vi "Find #SameModeChild.vi"(6 "Stop Traverse Child":bool, 8 "error in":errorcluster caption="错误输入（无错误）", 9 "Data in":cluster{"Split Mode":i32, "#sameMode":i32}={"Split Mode"=-1, "#sameMode"=0}, 11 "PanelRootNode.lvclass":refnum<class "PanelRootNode.lvclass">) -> (0 "error out":errorcluster caption="错误输出", 1 "Data out":cluster{"Split Mode":i32, "#sameMode":i32}, 3 "PanelRootNode.lvclass 2":refnum<class "PanelRootNode.lvclass">)   [LabVIEW 2013, in "PanelRootNode.lvclass"]
uses:
  PanelRootNode.lvclass
  PanelLinkNode/PanelLinkNode.lvclass/PanelLinkNode.ctl
  PanelLinkNode/PanelLinkNode.lvclass
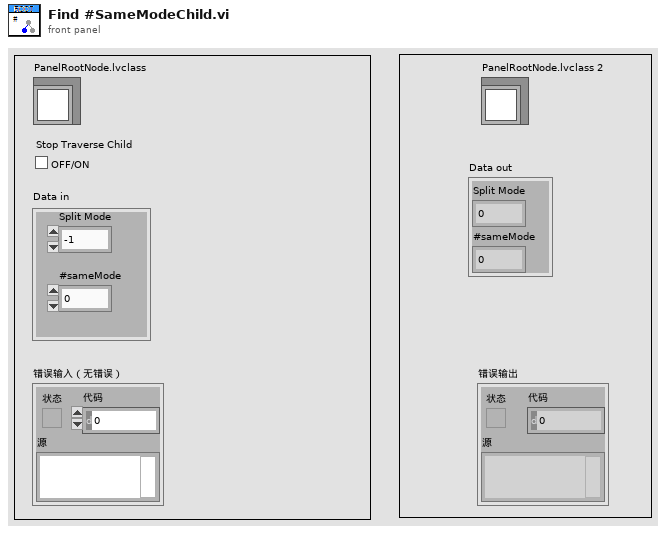
[diagram p1: front panel]
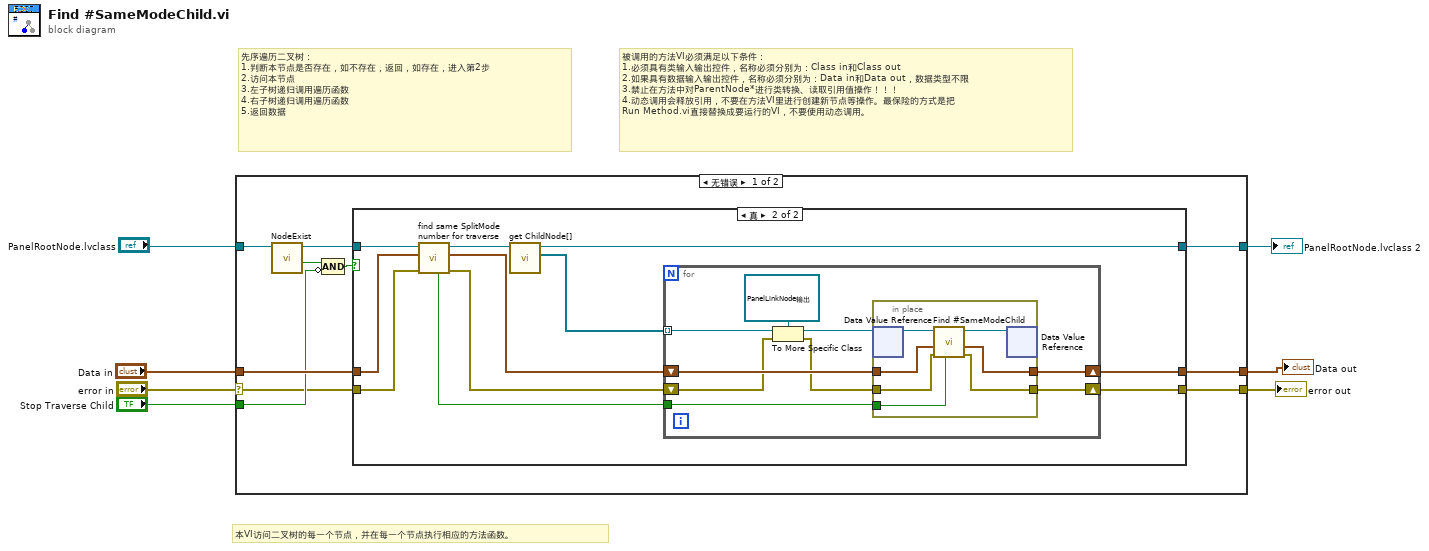
[diagram p0: block diagram]
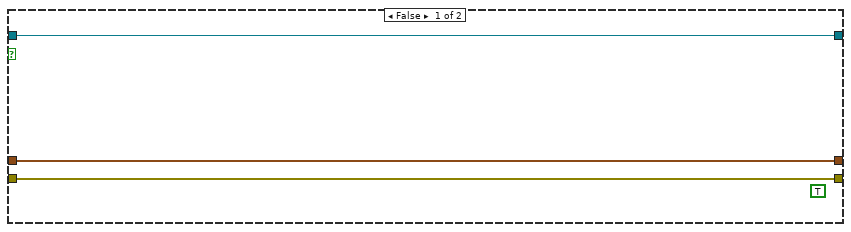
[diagram p2: hidden frame]
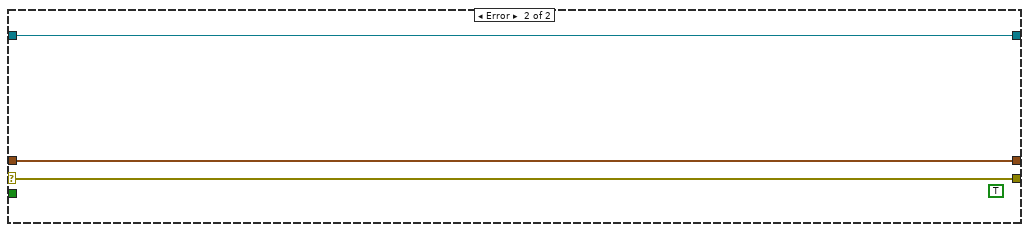
[diagram p3: hidden frame]
diagram:
  # "本VI访问二叉树的每一个节点，并在每一个节点执行相应的方法函数。"
  # "被调用的方法VI必须满足以下条件：\n1.必须具有类输入输出控件，名称必须分别为：Class in和Class out\n2.如果具有数据输入输出控件，名称必须分别为：Data in和Data out，数据类型不限\n3.禁止在方法中对ParentNode*进行类转换、读取引用值操作！！！\n4.动态调用会释放引用，不要在方法VI里进行创建新节点等操作。最保险的方式是把\nRun Method.vi直接替换成要运行的VI，不要使用动态调用。"
  # "先序遍历二叉树：\n1.判断本节点是否存在，如不存在，返回，如存在，进入第2步\n2.访问本节点\n3.左子树递归调用遍历函数\n4.右子树递归调用遍历函数\n5.返回数据"
  n1 = case shown="无错误" "error in" {
    selector: "error in" -> [w8 w50]
    tunnel: [w12 w50] -> w6
    tunnel: [w17 w49] -> w3
    tunnel: "PanelRootNode.lvclass" -> [w15 w49]
    tunnel: "Data in" -> [w16 w48]
    tunnel: [w13 w48] -> w1
    tunnel: "Stop Traverse Child" -> [w10 _]
    frame No Error {
      n2 = call-dynamic "NodeExist.vi"("PanelLinkNode 输入"=w15) -> ("Node Exist?"=w11:bool, "PanelLinkNode 输出"=w14:refnum<class "PanelRootNode.lvclass">)  [unwired: 8 in, 1 out]
      n3 = Compound Arithmetic op=AND(w11, invert w10) -> (w9:bool)
      n4 = case shown="真" w9 {
        tunnel: [w20 w23] -> w17
        tunnel: w16 -> [w19 w24]
        tunnel: w14 -> [w20 w29]
        tunnel: [w19 w21] -> w13
        tunnel: [w18 w31] -> w12
        tunnel: w8 -> [w18 w27]
        frame False {
          (unwired) TRUE ("Stop Traverse out")
        }
        frame True {
          n5 = call-dynamic "find same SplitMode number for traverse.vi"("error in (no error)"=w27, "Data in"=w24, "Class in"=w29) -> ("error out"=w26:errorcluster, "Data out"=w22:cluster{"Split Mode":i32, "#sameMode":i32}, "Class out"=w28:refnum<class "PanelRootNode.lvclass">, "Stop Traverse"=w25:bool)  [unwired: 5 in]
          n6 = call "get ChildNode[].vi"("PanelLinkNode输入"=w28) -> ("ChildNode*[]"=w30:refnum<data-value>[], "PanelLinkNode输出"=w23:refnum<class "PanelRootNode.lvclass">)  [unwired: 8 in, 1 out]
          n7 = for {
            tunnel: w30 -> [w40] mode=indexing
            shift-right: [w32] -> w31
            shift-left: w26 -> [w36]
            shift-right: [w33] -> w21
            shift-left: w22 -> [w38]
            tunnel: w25 -> [w37]
            n8 = To More Specific Class(target class=refnum<data-value> refnum ("数据值引用"), reference=w40, error in=w36) -> (specific class reference=w39:refnum<data-value>, error out=w35:errorcluster)
            n9 = in-place {
              in-place-border: w38 -> [w45]
              in-place-border: w35 -> [w44]
              in-place-border: w37 -> [w43]
              in-place-border: [w42] -> w33
              in-place-border: [w41] -> w32
              n10 = in-place-dvr #1(w39) -> (w47:refnum<class "PanelRootNode.lvclass">)  [unwired: 1 out]
              n11 = call "Find #SameModeChild.vi"("Stop Traverse Child"=w43, "error in"=w44, "Data in"=w45, "PanelRootNode.lvclass"=w47) -> ("error out"=w41:errorcluster, "Data out"=w42:cluster{"Split Mode":i32, "#sameMode":i32}, "PanelRootNode.lvclass 2"=w46:refnum<class "PanelRootNode.lvclass">)  [unwired: 5 in]
              n12 = in-place-dvr #1(w46) -> ()  [unwired: 2 out]
            }
          }
        }
      }
    }
    frame Error {
      (unwired) TRUE ("Stop Traverse out")
    }
  }
  "error out" <- w6
  "PanelRootNode.lvclass 2" <- w3
  "Data out" <- w1
